vi "save_pics.vi"(6 "name":string, 8 "error in (no error)":errorcluster, 9 "path":path, 10 "变体":variant, 11 "IMAQ image.ctl":T1) -> (0 "error out":errorcluster, 3 "identifying number":string)   [LabVIEW 2019]
uses:
  <vilib>/vision/Image Controls.llb/IMAQ Image.ctl
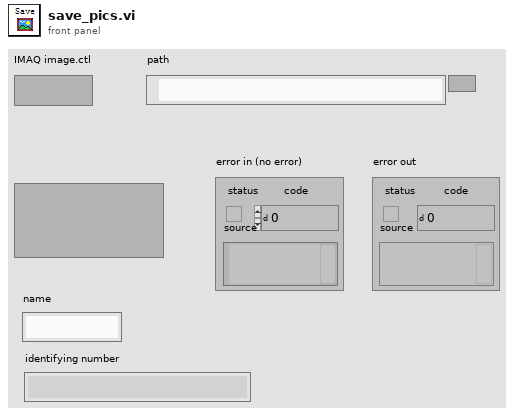
[diagram p1: front panel]
types:
  T1 = typedef "IMAQ Image.ctl" = refnum<image>
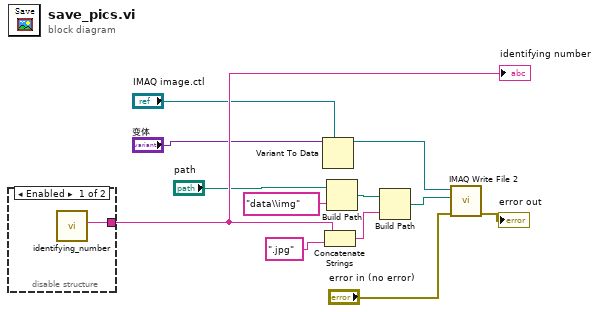
[diagram p0: block diagram]
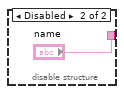
[diagram p2: hidden frame]
diagram:
  n1 = disable-structure shown="Enabled" {
    disable-tunnel: [w13 "name"] -> w7
    frame Enabled {
      n2 = call "identifying_number.vi"() -> ("identifying number"=w13:string)  [unwired: 11 in]
    }
    frame Disabled {
    }
  }
  "identifying number" <- w7
  n3 = Variant To Data(type="IMAQ image.ctl", Variant="变体") -> (data=w12:T1)  [unwired: 1 in, 1 out]
  n4 = Concatenate Strings(w7, ".jpg" ("字符串")) -> (w1:string)
  n5 = Build Path(base path="path", name or relative path="data\\img" ("名称或相对路径")) -> (appended path=w10:path)
  n6 = Build Path(base path=w10, name or relative path=w1) -> (appended path=w11:path)
  n7 = call-poly "IMAQ Write File 2"("error in (no error)"="error in (no error)", "File Path"=w11, "Image"=w12) -> ("error out"=→"error out":errorcluster)  [unwired: 7 in, 1 out]
